vi "VDH-markCalibrationStatus.vi"(11 "VDH-VNA_data_handler in":refnum<class "VDH-VNA_data_handler.lvclass">) -> (3 "VDH-VNA_data_handler out":refnum<class "VDH-VNA_data_handler.lvclass">)   [LabVIEW 2020, in "VDH-VNA_data_handler.lvlib" / "VDH-VNA_data_handler.lvclass"]
uses:
  VDH-VNA_data_handler.lvclass
  VDH-VNA_data_handler.lvclass/VDH-VNA_data_handler.ctl
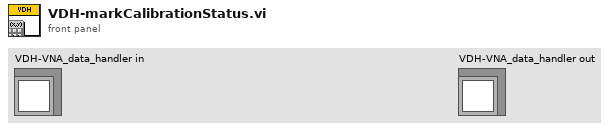
[diagram p1: front panel]
types:
  T1 = typedef "VDH-VNA_data_handler.lvlib/VDH-VNA_data_handler.lvclass/VDH-Calibration_enum.ctl" = enum16{"Non", "Short", "Open", "Load", "Through", "Permativity"}
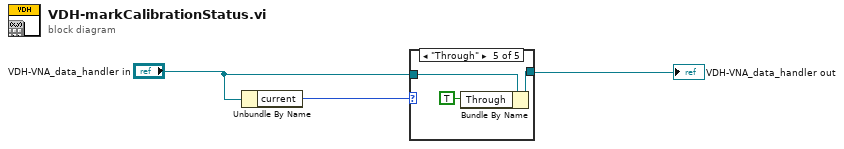
[diagram p0: block diagram]
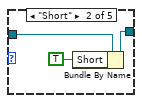
[diagram p3: hidden frame]
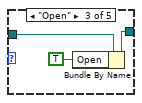
[diagram p4: hidden frame]
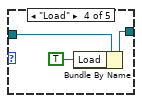
[diagram p5: hidden frame]
diagram:
  n1 = Unbundle By Name("VDH-VNA_data_handler in") -> ("current"=w1:T1)
  n2 = case shown="\"Through\"" w1 {
    tunnel: "VDH-VNA_data_handler in" -> [w4 w7 w10 w13 w16]
    tunnel: [w4 w6 w9 w12 w15] -> w2
    frame "Non", Default {
    }
    frame "Short" {
      n3 = Bundle By Name(cluster=w7, "Short"=TRUE ("Calibration Status.Calib Status.Short")) -> (w6:refnum<class "VDH-VNA_data_handler.lvclass">)
    }
    frame "Open" {
      n4 = Bundle By Name(cluster=w10, "Open"=TRUE ("Calibration Status.Calib Status.Short")) -> (w9:refnum<class "VDH-VNA_data_handler.lvclass">)
    }
    frame "Load" {
      n5 = Bundle By Name(cluster=w13, "Load"=TRUE ("Calibration Status.Calib Status.Short")) -> (w12:refnum<class "VDH-VNA_data_handler.lvclass">)
    }
    frame "Through" {
      n6 = Bundle By Name(cluster=w16, "Through"=TRUE ("Calibration Status.Calib Status.Short")) -> (w15:refnum<class "VDH-VNA_data_handler.lvclass">)
    }
  }
  "VDH-VNA_data_handler out" <- w2
